vi "subStage_GetPosition.vi"(7 "Stage Info In":T1={" Current Position"=[-1.0, -12.0, 0.0], "Number of Axis"=3, "ILSID"=1}, 8 "Error In":errorcluster) -> (0 "Error out":errorcluster, 5 "Stage Info Out":T1={" Current Position"=[-1.0, -12.0, 0.0], "Number of Axis"=3, "ILSID"=1})   [LabVIEW 2015]
panel:
  # "X"
  # "Y"
  # "X"
  # "Y"
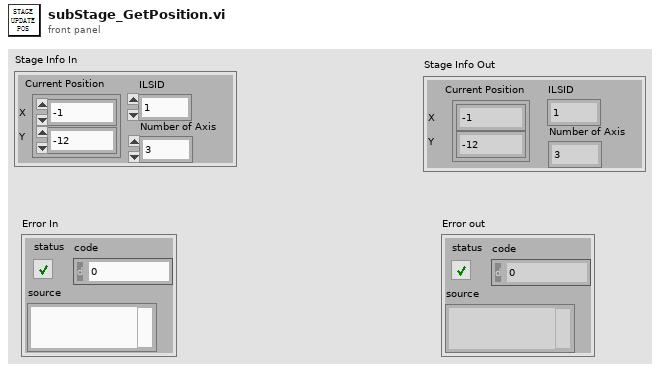
[diagram p1: front panel]
types:
  T1 = cluster{" Current Position":dbl[], "Number of Axis":i32, "ILSID":i32}
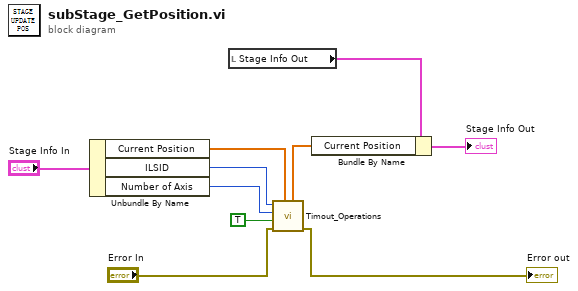
[diagram p0: block diagram]
diagram:
  n1 = Unbundle By Name("Stage Info In") -> ("Current Position"=w4:dbl[], "ILSID"=w5:i32, "Number of Axis"=w6:i32)
  n2 = local read "Stage Info Out"() -> (w2:T1)
  n3 = call "Timout_Operations.vi"("PosIn"=w4, "Error In"="Error In", "Connected?"=TRUE, "Number Of Axes"=w6, "lLSID"=w5) -> ("Error out"=→"Error out":errorcluster, "PosOut"=w3:dbl[])  [unwired: 2 in, 3 out]
  n4 = Bundle By Name(cluster=w2, "Current Position"=w3) -> (→"Stage Info Out":T1)
